vi "TestExec.Sequence, Populate Variables.vi"(8 "error in":errorcluster, 10 "Variable Values":variant, 11 "Param In":string) -> (0 "error out":errorcluster, 3 "Param Out":string)   [LabVIEW 2018]
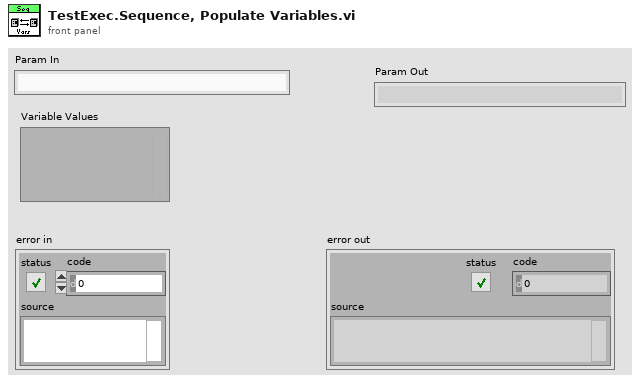
[diagram p1: front panel]
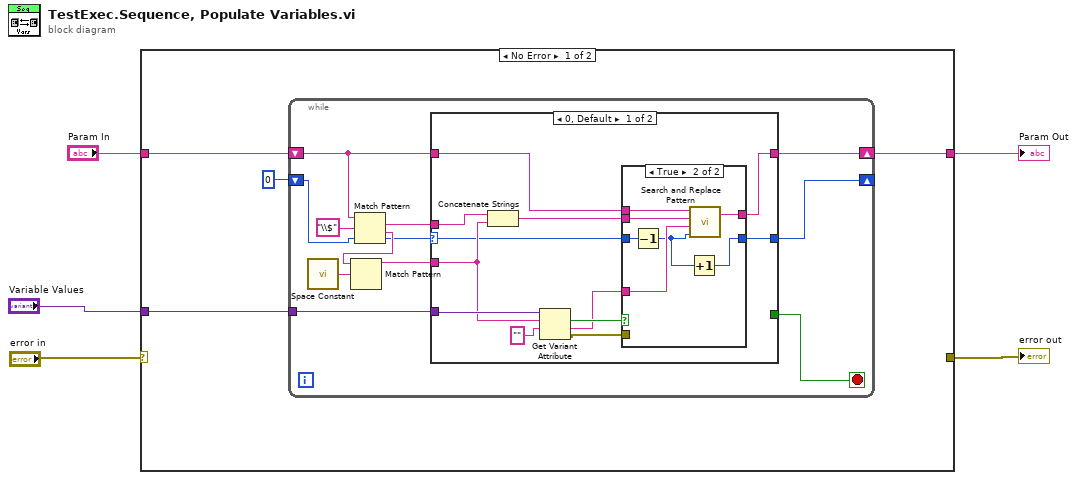
[diagram p0: block diagram]
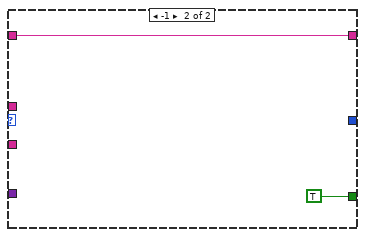
[diagram p3: hidden frame]
diagram:
  n1 = case shown="No Error" "error in" {
    selector: "error in" -> [_ w45]
    tunnel: [w9 w46] -> w5
    tunnel: "Param In" -> [w8 w46]
    tunnel: [_ w45] -> w2
    tunnel: "Variable Values" -> [w6 _]
    frame No Error {
      n2 = while {
        shift-right: [w14] -> w9
        shift-left: w8 -> [w15]
        tunnel: w6 -> [w12]
        shift-right: [w10] -> _
        shift-left: 0 -> [w11]
        stop <- w16 stop-if-true
        n3 = call <vilib>:"Space Constant.vi"() -> ("String"=w19:string)
        n4 = Match Pattern(string=w15, regular expression="\\$", offset (0)=w11) -> (match substring=w13:string, after substring=w20:string, offset past match=w18:i32)  [unwired: 1 out]
        n5 = Match Pattern(string=w20, regular expression=w19) -> (before substring=w17:string)  [unwired: 1 in, 3 out]
        n6 = case shown="0, Default" w18 {
          selector: w18 -> [w23 _]
          tunnel: w17 -> [w28 _]
          tunnel: [_ TRUE] -> w16
          tunnel: w15 -> [w32 w43]
          tunnel: [w31 w43] -> w14
          tunnel: w13 -> [w33 _]
          tunnel: w12 -> [w29 _]
          tunnel: [w22 _] -> w10
          frame 0, Default {
            n7 = Concatenate Strings(w33, w28) -> (w30:string)
            n8 = Get Variant Attribute(Variant=w29, name=w28, default value (empty Variant)="") -> (found=w27:bool, value=w24:string, error out=w26:errorcluster)  [unwired: 1 in, 1 out]
            n9 = case shown="True" w27 {
              tunnel: w32 -> [w35 w42]
              tunnel: [w35 w41] -> w31
              tunnel: w30 -> [_ w40]
              tunnel: w26 -> [_ _]
              tunnel: w24 -> [_ w39]
              tunnel: w23 -> [w34 w37]
              tunnel: [w34 w38] -> w22
              frame False {
              }
              frame True {
                n10 = Decrement(x=w37) -> (x-1=w36:i32)
                n11 = Increment(x=w36) -> (x+1=w38:i32)
                n12 = call <vilib>:"Search and Replace Pattern.vi"("string"=w42, "regular expression (\"\")"=w40, "replace string (\"\")"=w39, "offset (0)"=w36) -> ("result string"=w41:string)  [unwired: 1 in, 1 out]
              }
            }
          }
          frame -1 {
          }
        }
      }
    }
    frame Error {
    }
  }
  "error out" <- w2
  "Param Out" <- w5
